vi "CryoCooler GUI.vi"(9 "Standalone":bool=TRUE, 10 "Init Data":variant, 11 "CryoCooler Name":string) -> ()   [LabVIEW 2024]
uses:
  typedefs/CC enum Operation Mode.ctl
  Cryo Cooler/CryoCoolerAVC/CryoCoolerAVC Command enum.ctl
  Subsystems/SS typedef cluster Instrument Command Queue Data.ctl
  Subsystems/SS cluster Data Queue type.ctl
  hk-channel-class/hk-channel-class/HK Item/HK Item.lvclass
  Cryo Cooler/Cryo Cooler.lvclass
  Cryo Cooler/CryoCoolerAVC/CryoCoolerAVC Command cluster.ctl
  typedefs/CC cluster Alarm Data.ctl
  CryoCooler cluster Alarm Settings.ctl
  Power Distribution/Power Distribution.lvclass
  typedefs/CC cluster Outlet Control.ctl
  typedefs/CC enum Status FG Action.ctl
  Cryo Cooler/CryoCoolerAVC/CryoCoolerAVC.lvclass
  typedefs/CC enum Subsystem Status.ctl
  hk-channel-class/hk-channel-class/HK Item/HK Item.lvclass/HK Item.ctl
  Power Distribution/Orion PDU/Orion PDU.lvclass
  hk-channel-class/hk-channel-class/HK Item/HK Channel cluster Telemetry Data.ctl
  hk-channel-class/hk-channel-class/HK Item/HK Channel enum Data Type.ctl
  <vilib>/Utility/error.llb/DialogType.ctl
  hk-channel-class/hk-channel-class/HK Item/Write Source.vi
  6db094d1-7fd6-4988-9962-decbce56bcaa.vi
  40afddd7-fa93-47ab-b467-3e4868690066.vi
panel:
  in  "Mode":T1
  in  "Tab Control":T2(tab)
  out "Alarm Message":string
  out "Cryo Connected":bool
  out "Alarm":bool
  in  "Status":i32[](listbox)
  out "XY Graph":T3(graph)
  out "Cryo 2":bool
  out "Cryo 1":bool
  in  "Configure Alarms":bool
  in  "Select Cryo Cooler":u16(ring) items=["Cooler1", "Cooler2", "Cooler3"]
  in  "Shutdown Temp":dbl caption="Reject Temp Shutdown Temp"
  in  "Init Message":string="Connecting to Hardware..."
  in  "Reinit":bool
  out "Response":string[](array[string])
  in  "Execute command":bool
  in  "Command Options":string="On"
  in  "Command":T4=1 items=["STATUS", "COOLER", "E", "ERROR", "KD", "KI", "KP", "LOGIN", "LOGOUT", "MODE", "P", "PWOUT", "SENSOR", "TC", "TEMP RJ", "TTARGET", "VERSION"]
  in  "Address":refnum<visa-resource-name>
  in  "CryoCooler Type":u16(ring) items=["Simulation", "RIMAS"]
  in  "Close":bool
  out "x-y":u32
  in  "Simulate":bool
  out "Current 2":dbl caption="Current" format="%_3g"
  out "Current":dbl format="%_3g"
  in  "Settings Button 2":bool
  in  "Refresh Button 2":bool
  in  "Names 2":string[](array[string])=["OutletA", "OutletB", "Lshore325", "Lshore218", "Lshore331", "PfeifferG", "Comms", "Motor"] caption="Names"
  in  "Relay Set 2":bool[](array[boolean]) caption="Set"
  out "Status 2":bool[](array[boolean]) caption="Status"
  in  "Settings Button":bool
  in  "Names":string[](array[string])=["MACIE", "Cryo1_3", "Cryo2", "Lesker", "Hg Argon", "Krypton", "Mercury", "Xenon"]
  in  "Relay Set":bool[](array[boolean]) caption="Set"
  out "Status":bool[](array[boolean])
  in  "Refresh Button":bool
  out "Log":string
  in  "Cryo 1 Pwr":bool
  in  "Cryo 2 Pwr":bool
  # "PDU 1"
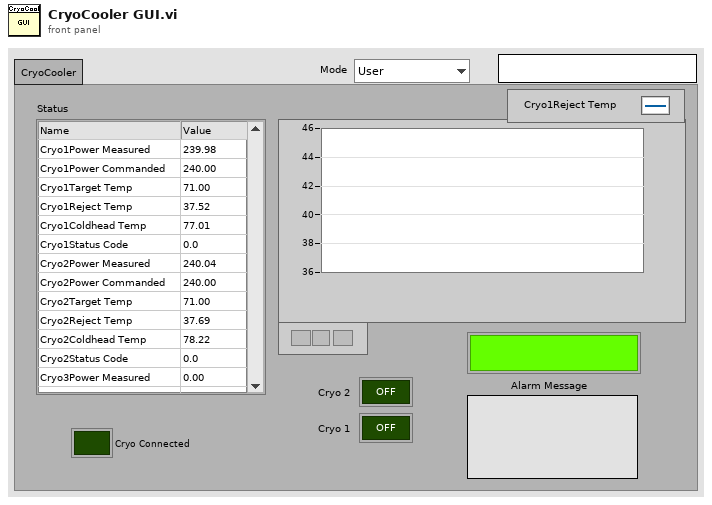
[diagram p1: front panel]
types:
  T1 = typedef "CC enum Operation Mode.ctl" = enum16{"User", "Engineering"}
  T2 = enum32{"CryoCooler", "Engineering", "Power", "Log"}
  T3 = cluster{cluster{"Time Stamp":timestamp, "Numeric":dbl}[]}[]
  T4 = typedef "CryoCoolerAVC.lvclass/CryoCoolerAVC Command enum.ctl" = u16
  T5 = typedef "SS typedef cluster Instrument Command Queue Data.ctl" = cluster{"Cmd":string, "Parameters":variant}
  T6 = typedef "CryoCoolerAVC.lvclass/CryoCoolerAVC Command cluster.ctl" = cluster{"Command":T4, "Options":string, "Cryo Idx":i32}
  T7 = typedef "CC cluster Alarm Data.ctl" = cluster{"Measured Value":dbl, "Alarm Low":dbl, "Alarm High":dbl, "Message":string, "Source":string}
  T8 = typedef "CryoCooler cluster Alarm Settings.ctl" = cluster{"Reject Shutdown Temp":dbl, "Reject Temp Warning":dbl, "Temperature Error Max":dbl, "Enabled":bool}
  T9 = typedef "CC cluster Outlet Control.ctl" = cluster{"Outlet Idx":i32, "State":bool}
  T10 = cluster{"state":refnum<user-event>, "cmd q":refnum<queue>, "Cmd":T5, "Data Q":refnum<queue>, "error":errorcluster, "next poll":timestamp, "Cryo Name":string, "poll":bool, "Channel List":refnum<class "HK Item.lvclass">[], "Focus Pos":dbl, "Cryo Cooler ref":refnum<class "Cryo Cooler.lvclass">, "Data":dbl[], "Cryo Cmd":T6, "Alarm":bool, "Alarms":T7[], "Source":string, "Cryo Alarms":T8, "Shutdown":bool, "Relays Enable":bool, "PDUs":refnum<class "Power Distribution.lvclass">[], "outlet":T9}
  T11 = typedef "CC enum Status FG Action.ctl" = enum16{"Read", "Write", "Init"}
  T12 = typedef "CC enum Subsystem Status.ctl" = enum16{"Unknown", "Ready", "Error"}
  T13 = typedef "SS cluster Data Queue type.ctl" = cluster{"Source":string, "Type":string, "Data":variant}
  T14 = typedef "HK Item.lvclass/HK Channel enum Data Type.ctl" = enum16{"Floating Point", "Integer", "Enum", "String", "Waveform", "File"}
  T15 = typedef "HK Item.lvclass/HK Channel cluster Telemetry Data.ctl" = cluster{"Ch Names":string[], "Ch Values":dbl[], "Timestamp":timestamp, "Data Type":T14}
  T16 = typedef "CC cluster Device Index.ctl" = cluster{"Device Type Name":string, "Curr Device Name":string, "All Instances":string[]}
  T17 = typedef "CryoCooler Default User Settings.ctl" = cluster{"Select Ch":i32[], "Default Device":string}
  T18 = typedef "CryoCoolerAVC.lvclass/CryoCoolerAVC Settings.ctl" = cluster{"Cryo Addr":refnum<visa-resource-name>[]}
  T19 = typedef "HK Item.lvclass/HK Channel Units and Setup.ctl" = cluster{"Unit Type":string, "Units":string, "Configuration":string, "Digits":i32, "Data Type":T14, "Exponential?":bool, "Source":string}
  T20 = cluster{"[0]":dbl, "[1]":dbl, "[2]":dbl, "[3]":dbl, "[4]":dbl, "[5]":dbl}[]
  T21 = cluster{cluster{"Time Stamp":timestamp, "Numeric":dbl}[]}
  T22 = typedef "DialogType.ctl" = u16
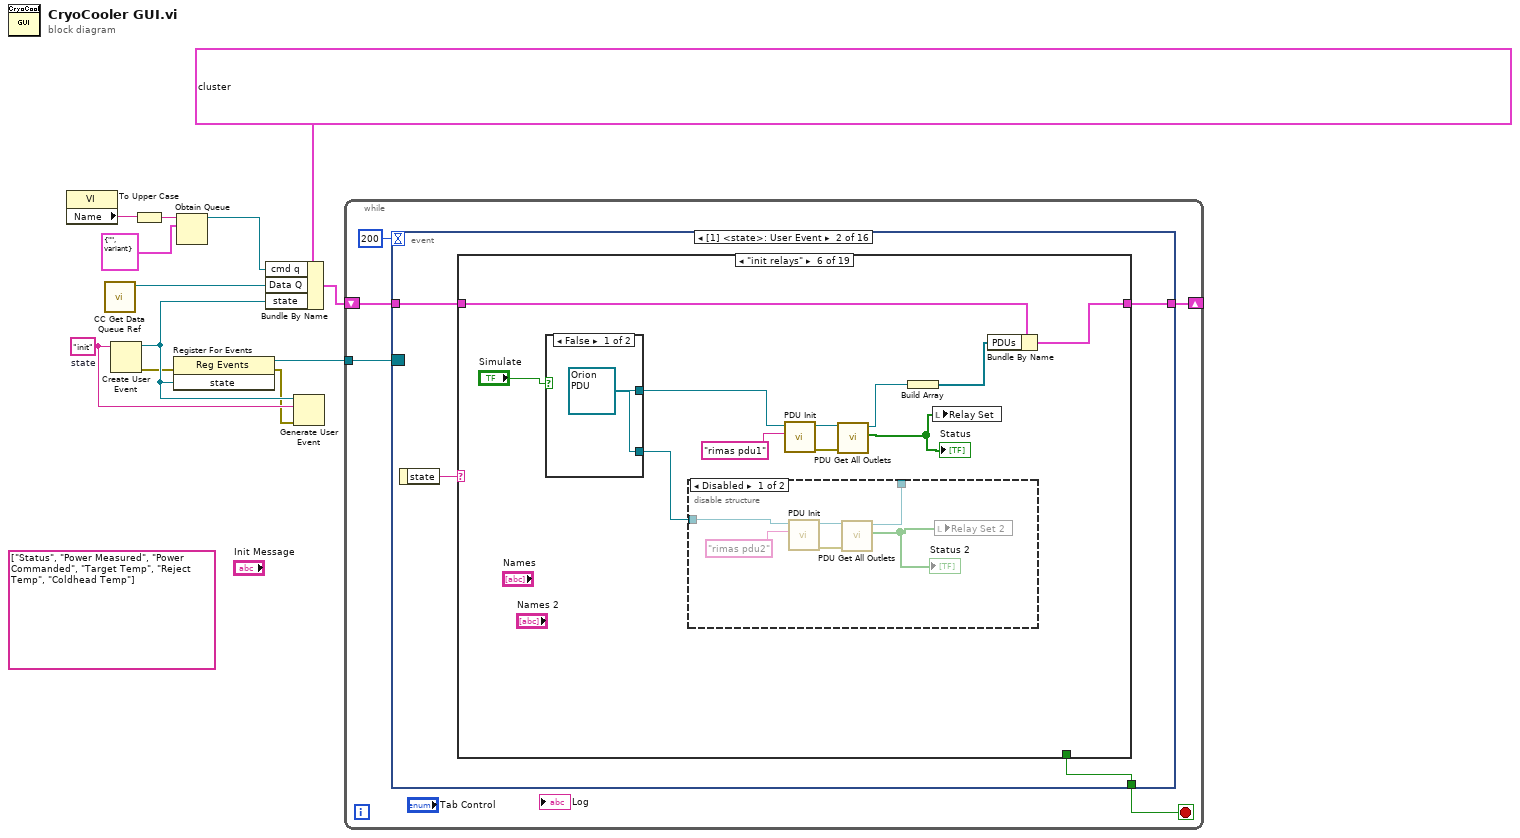
[diagram p0: block diagram]
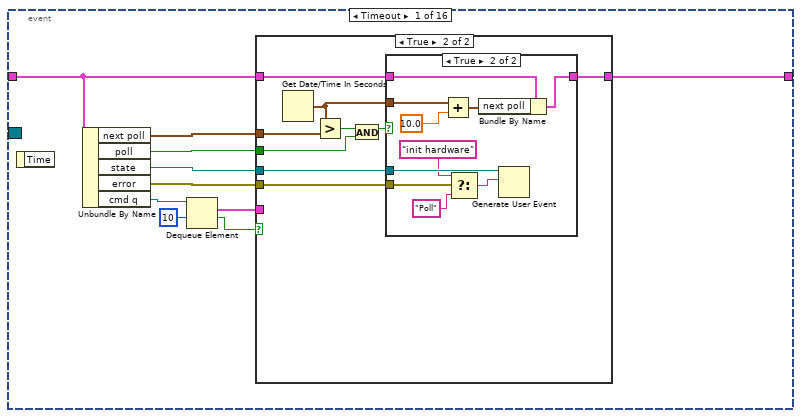
[diagram p2: hidden frame]
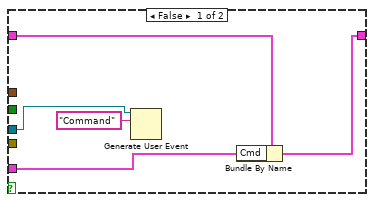
[diagram p3: hidden frame]
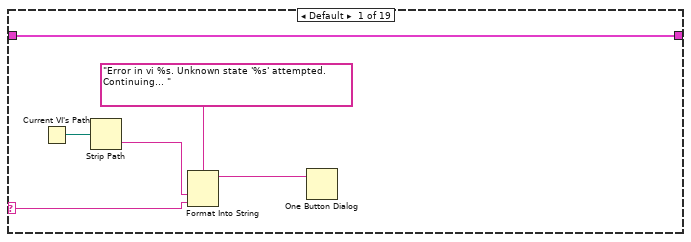
[diagram p5: hidden frame]
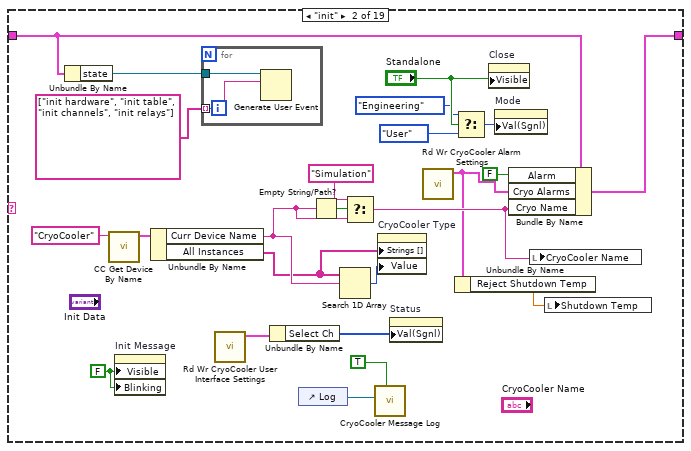
[diagram p6: hidden frame]
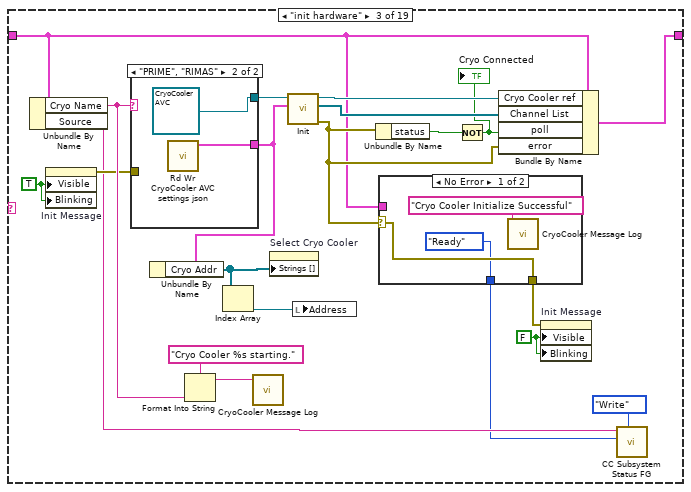
[diagram p7: hidden frame]
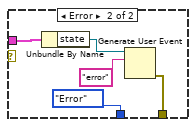
[diagram p8: hidden frame]
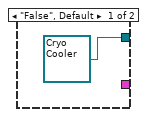
[diagram p9: hidden frame]
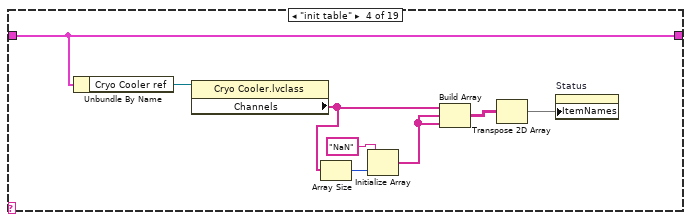
[diagram p10: hidden frame]
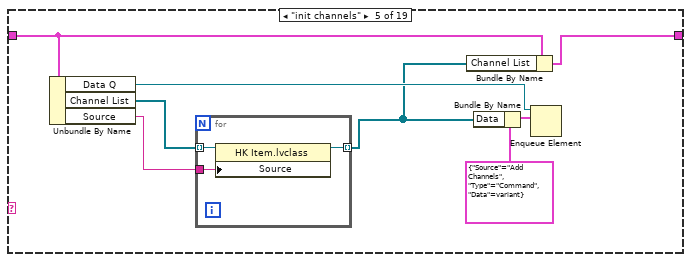
[diagram p11: hidden frame]
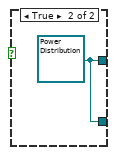
[diagram p13: hidden frame]
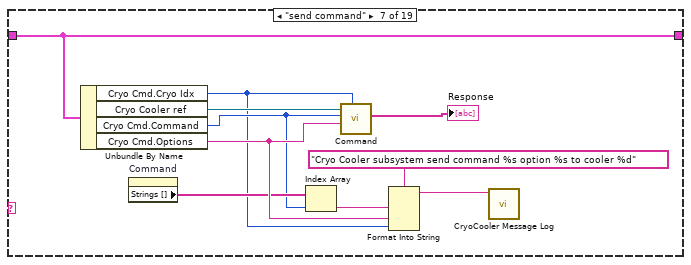
[diagram p14: hidden frame]
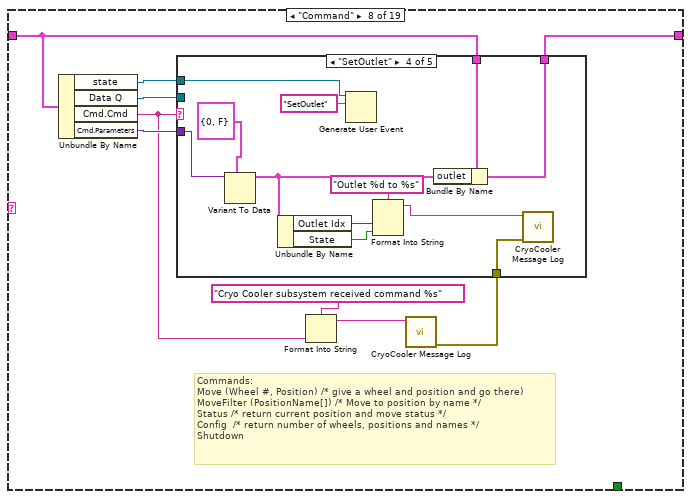
[diagram p15: hidden frame]
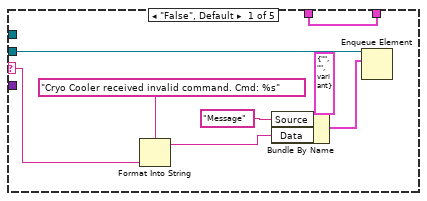
[diagram p16: hidden frame]
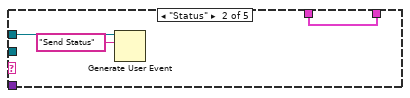
[diagram p17: hidden frame]
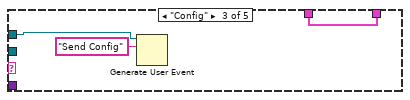
[diagram p18: hidden frame]
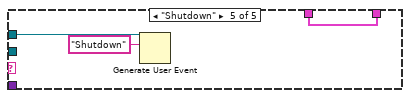
[diagram p19: hidden frame]
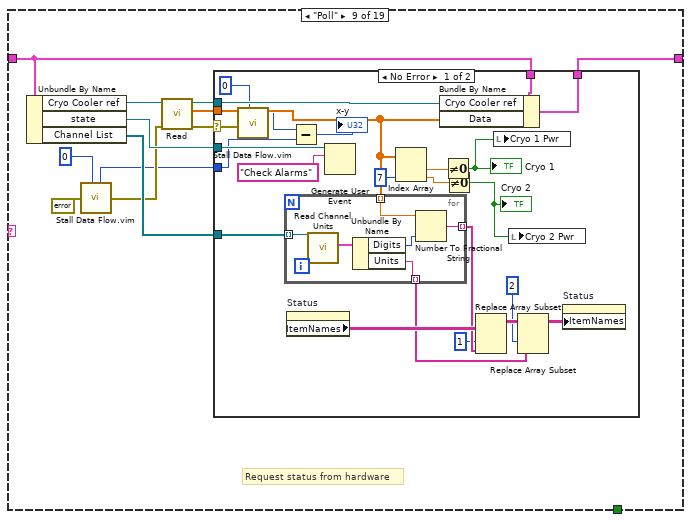
[diagram p20: hidden frame]
diagram:
  (unwired) string[] ["Status", "Power Measured", "Power Commanded", "Target Temp", "Reject Temp", "Coldhead Temp"]
  w8 = "init"  # state
  n1 = property class="VI"() -> ("Name"=w4:string)  [unwired: 2 in, 2 out]
  n2 = call "CC Get Data Queue Ref.vi"() -> ("Data Q"=w5:refnum<queue>)  [unwired: 10 in, 1 out]
  n3 = Create User Event(user event datatype=w8) -> (user event=w10:refnum<user-event>, error out=w6:errorcluster)  [unwired: 1 in]
  n4 = To Upper Case(1:w4) -> (0:w3:string)
  n5 = register-events(error in=w6, w10) -> (reference out=w9:refnum<event-registration>, error out=w7:errorcluster)  [unwired: 1 in]
  n6 = Obtain Queue(name (unnamed)=w3, element data type=T5 {"Cmd"="", "Parameters"=variant}) -> (queue out=w1:refnum<queue>)  [unwired: 3 in, 2 out]
  n7 = Bundle By Name(cluster=T10 {"state"=refnum, "cmd q"=refnum, "Cmd"={"Cmd"="", "Parameters"=variant}, "Data Q"=refnum, "error"={"status"=FALSE, "code"=0, "source"=""}, "next poll"=timestamp(0 s since 1904-01-01), "Cryo Name"="", "poll"=FALSE, "Channel List"=[], "Focus Pos"=0.0, "Cryo Cooler ref"=refnum, "Data"=[], "Cryo Cmd"={"Command"=0, "Options"="", "Cryo Idx"=0}, "Alarm"=FALSE, "Alarms"=[], "Source"="CryoCooler", "Cryo Alarms"={"Reject Shutdown Temp"=30.0, "Reject Temp Warning"=3.0, "Temperature Error Max"=60.0, "Enabled"=FALSE}, "Shutdown"=FALSE, "Relays Enable"=FALSE, "PDUs"=[], "outlet"={"Outlet Idx"=0, "State"=FALSE}}, "cmd q"=w1, "Data Q"=w5, "state"=w10) -> (w11:T10)
  n8 = Generate User Event(user event=w10, event data cluster=w8, error in=w7) -> ()  [unwired: 1 in, 2 out]
  n9 = while {
    tunnel: w9 -> [w17]
    shift-right: [w15] -> _
    shift-left: w11 -> [w16]
    stop <- w14 stop-if-true
    n10 = event shown="[1] <state>: User Event" {
      selector: w17 -> [_ _ _ _ _ _ _ _ _ _ _ _ _ _ _ _]
      dyn-events: _ -> [_ _ _ _ _ _ _ _ _ _ _ _ _ _ _ _]
      timeout: 200 -> [_ _ _ _ _ _ _ _ _ _ _ _ _ _ _ _]
      tunnel: w16 -> [w22 w55 w382 w397 w401 w409 w415 w425 w437 w451 w453 w459 w467 w473 w492 w499]
      tunnel: [w21 w54 w383 w398 w402 w407 w415 w425 w438 w451 w453 w460 w467 w474 w492 w499] -> w15
      tunnel: [_ w53 _ _ _ _ _ _ _ _ _ _ _ _ _ _] -> w14
      event Timeout {
        n11 = event-data() -> ()  [unwired: 1 in, 1 out]
        n12 = Unbundle By Name(w22) -> ("next poll"=w20:timestamp, "poll"=w19:bool, "state"=w23:refnum<user-event>, "error"=w18:errorcluster, "cmd q"=w27:refnum<queue>)
        n13 = Dequeue Element(queue=w27, timeout in ms (-1)=10) -> (element=w24:T5, timed out?=w25:bool)  [unwired: 1 in, 2 out]
        n14 = case shown="True" w25 {
          tunnel: w24 -> [w29 _]
          tunnel: w23 -> [w32 w38]
          tunnel: w22 -> [w30 w39]
          tunnel: [w28 w36] -> w21
          tunnel: w20 -> [_ w41]
          tunnel: w19 -> [_ w34]
          tunnel: w18 -> [_ w33]
          frame False {
            n15 = Generate User Event(user event=w32, event data cluster="Command" ("event data")) -> ()  [unwired: 2 in, 2 out]
            n16 = Bundle By Name(cluster=w30, "Cmd"=w29) -> (w28:T10)
          }
          frame True {
            n17 = Get Date/Time In Seconds() -> (seconds since 1Jan1904=w37:timestamp)
            n18 = Greater?(x=w37, y=w41) -> (0:w40:bool)
            n19 = And(x=w40, y=w34) -> (x .and. y?=w35:bool)
            n20 = case shown="True" w35 {
              tunnel: w39 -> [w42 w52]
              tunnel: w38 -> [_ w51]
              tunnel: w37 -> [_ w50]
              tunnel: [w42 w47] -> w36
              tunnel: w33 -> [_ w45]
              frame False {
              }
              frame True {
                n21 = Add(x=w50, y=10.0) -> (x+y=w48:timestamp)
                n22 = Select(t="init hardware", s=w45, f="Poll" ("event data")) -> (s? t:f=w43:string)
                n23 = Bundle By Name(cluster=w52, "next poll"=w48) -> (w47:T10)
                n24 = Generate User Event(user event=w51, event data cluster=w43) -> ()  [unwired: 2 in, 2 out]
              }
            }
          }
        }
      }
      event User Event {
        n25 = event-data() -> ("state"=w56:string)  [unwired: 1 in]
        n26 = case shown="\"init relays\"" w56 {
          selector: w56 -> [w61 _ _ _ _ _ _ _ _ _ _ _ _ _ _ _ _ _ _]
          tunnel: w55 -> [w57 w84 w100 w128 w130 w148 w167 w173 w217 w266 w280 w284 w297 w305 w317 w335 w339 w346 w371]
          tunnel: [w57 w85 w109 w128 w131 w150 w167 w174 w218 w267 w280 w285 w297 w305 w317 w335 w340 w347 w371] -> w54
          tunnel: [_ _ _ _ _ _ _ _ _ _ _ _ _ _ _ _ _ _ TRUE] -> w53
          frame Default {
            n27 = Current VI's Path() -> (path=w60:path)
            n28 = Strip Path(path=w60) -> (name=w59:string)  [unwired: 1 out]
            n29 = Format Into String(format string="Error in vi %s. Unknown state '%s' attempted. Continuing... ", w59, w61) -> (resulting string=w58:string)  [unwired: 2 in, 1 out]
            n30 = One Button Dialog(message=w58) -> ()  [unwired: 1 in, 1 out]
          }
          frame "init" {
            w66 = FALSE ("Visible")
            n31 = Unbundle By Name(w84) -> ("state"=w83:refnum<user-event>)
            n32 = call "CC Get Device By Name.vi"("Device Type"="CryoCooler") -> ("Device"=w78:T16)  [unwired: 8 in, 2 out]
            n33 = property on="Init Message" class="Str"("Visible"=w66, "Blinking"=w66) -> ()  [unwired: 2 in, 2 out]
            n34 = Unbundle By Name(w78) -> ("Curr Device Name"=w77:string, "All Instances"=w76:string[])
            n35 = for {
              tunnel: w83 -> [w88]
              tunnel: string[] ["init hardware", "init table", "init channels", "init relays"] -> [w87] mode=indexing
              n36 = Generate User Event(user event=w88, event data cluster=w87) -> ()  [unwired: 2 in, 2 out]
            }
            n37 = call "Rd Wr CryoCooler User Interface Settings.vi"() -> ("Settings"=w71:T17)  [unwired: 10 in, 1 out]
            n38 = Unbundle By Name(w71) -> ("Select Ch"=w70:i32[])
            n39 = control-ref of="Log"() -> (w69:refnum<vi>)
            n40 = Empty String/Path?(string/path=w77) -> (empty?=w86:bool)
            n41 = Search 1D Array(1D array=w76, element=w77) -> (index of element=w81:i32)  [unwired: 1 in]
            n42 = Select(t="Simulation", s=w86, f=w77) -> (s? t:f=w67:string)
            n43 = call "CryoCooler Message Log.vi"("init?"=TRUE, "Log Ref"=w69) -> ()  [unwired: 8 in, 2 out]
            n44 = property on="CryoCooler Type" class="Ring (strict)"("Strings []"=w76, "Value"=w81) -> ()  [unwired: 2 in, 2 out]
            n45 = property on="Status" class="MCListbox (strict)"("Val(Sgnl)"=w70) -> ()  [unwired: 2 in, 2 out]
            n46 = call "Rd Wr CryoCooler Alarm Settings.vi"() -> ("Cryo Alarms out"=w65:T8)  [unwired: 10 in, 1 out]
            n47 = Unbundle By Name(w65) -> ("Reject Shutdown Temp"=w64:dbl)
            n48 = Select(t=CC_enum_Operation_Mode."Engineering" ("Mode"), s="Standalone", f=CC_enum_Operation_Mode."User" ("Mode")) -> (s? t:f=w72:T1)
            n49 = property on="Close" class="Bool"("Visible"="Standalone") -> ()  [unwired: 2 in, 2 out]
            n50 = property on="Mode" class="Enum (strict)"("Val(Sgnl)"=w72) -> ()  [unwired: 2 in, 2 out]
            n51 = Bundle By Name(cluster=w84, "Alarm"=FALSE, "Cryo Alarms"=w65, "Cryo Name"=w67) -> (w85:T10)
            n52 = local write "CryoCooler Name"(w67) -> ()
            n53 = local write "Shutdown Temp"(w64) -> ()
          }
          frame "init hardware" {
            w95 = FALSE ("Visible")
            w97 = TRUE ("Visible")
            n54 = Unbundle By Name(w100) -> ("Cryo Name"=w104:string, "Source"=w92:string)
            n55 = property on="Init Message" class="Str"("Visible"=w97, "Blinking"=w97) -> (error out=w96:errorcluster)  [unwired: 2 in, 1 out]
            n56 = case shown="\"PRIME\", \"RIMAS\"" w104 {
              tunnel: [refnum<class "Cryo Cooler.lvclass"> refnum ("Cryo Cooler.lvclass") refnum<class "CryoCoolerAVC.lvclass"> refnum ("CryoCoolerAVC.lvclass")] -> w106
              tunnel: [_ w119] -> w103
              tunnel: w96 -> [_ _]
              frame "False", Default {
              }
              frame "PRIME", "RIMAS" {
                n57 = call "Rd Wr CryoCooler AVC settings json.vi"() -> ("CryoCooler Settings"=w119:T18)  [unwired: 10 in, 1 out]
              }
            }
            n58 = Unbundle By Name(w103) -> ("Cryo Addr"=w90:refnum<visa-resource-name>[])
            n59 = Format Into String(format string="Cryo Cooler %s starting.", w104) -> (resulting string=w98:string)  [unwired: 2 in, 1 out]
            n60 = Index Array(array=w90) -> (element=w89:refnum<visa-resource-name>)  [unwired: 1 in]
            n61 = call "CryoCooler Message Log.vi"("String in"=w98) -> ()  [unwired: 9 in, 2 out]
            n62 = property on="Select Cryo Cooler" class="Ring (strict)"("Strings []"=w90) -> ()  [unwired: 2 in, 2 out]
            n63 = call-dynamic "Init.vi"("Init Data"=w103, "Cryo Cooler in"=w106) -> ("error out"=w101:errorcluster, "Channel List"=w105:refnum<class "HK Item.lvclass">[], "Cryo Cooler out"=w107:refnum<class "Cryo Cooler.lvclass">)  [unwired: 7 in]
            n64 = local write "Address"(w89) -> ()
            n65 = Unbundle By Name(w101) -> ("status"=w108:bool)
            n66 = case shown="No Error" w101 {
              selector: w101 -> [w111 _]
              tunnel: w100 -> [_ w117]
              tunnel: [w111 w114] -> w94
              tunnel: [CC_enum_Subsystem_Status."Ready" ("Status") CC_enum_Subsystem_Status."Error" ("Status")] -> w91
              frame No Error {
                n67 = call "CryoCooler Message Log.vi"("String in"="Cryo Cooler Initialize Successful") -> ()  [unwired: 9 in, 2 out]
              }
              frame Error {
                n68 = Unbundle By Name(w117) -> ("state"=w116:refnum<user-event>)
                n69 = Generate User Event(user event=w116, event data cluster="error" ("event data")) -> (error out=w114:errorcluster)  [unwired: 2 in, 1 out]
              }
            }
            n70 = Not(x=w108) -> (.not. x?=w99:bool)
            "Cryo Connected" <- w99
            n71 = Bundle By Name(cluster=w100, "Cryo Cooler ref"=w107, "Channel List"=w105, "poll"=w99, "error"=w101) -> (w109:T10)
            n72 = property on="Init Message" class="Str"(error in=w94, "Visible"=w95, "Blinking"=w95) -> ()  [unwired: 1 in, 2 out]
            n73 = call "CC Subsystem Status FG.vi"("Action"=CC_enum_Status_FG_Action."Write", "Status"=w91, "Subsystem Name"=w92) -> ()  [unwired: 7 in, 2 out]
          }
          frame "init table" {
            n74 = Unbundle By Name(w128) -> ("Cryo Cooler ref"=w127:refnum<class "Cryo Cooler.lvclass">)
            n75 = property class="Cryo Cooler.lvclass"(reference=w127) -> ("Channels"=w125:string[])  [unwired: 1 in, 2 out]
            n76 = Array Size(array=w125) -> (size(s)=w126:i32)
            n77 = Initialize Array("NaN", w126) -> (w121:string[])
            n78 = Build Array(w125, w121, w121) -> (w123:string[][])
            n79 = Transpose 2D Array(2D array=w123) -> (transposed array=w122:string[][])
            n80 = property on="Status" class="MCListbox (strict)"("ItemNames"=w122) -> ()  [unwired: 2 in, 2 out]
          }
          frame "init channels" {
            n81 = Unbundle By Name(w130) -> ("Data Q"=w134:refnum<queue>, "Channel List"=w133:refnum<class "HK Item.lvclass">[], "Source"=w129:string)
            n82 = for {
              tunnel: w133 -> [w139] mode=indexing
              tunnel: [w138] -> w132 mode=indexing
              tunnel: w129 -> [w137]
              n83 = property class="HK Item.lvclass"(reference=w139, "Source"=w137) -> (reference out=w138:refnum<class "HK Item.lvclass">)  [unwired: 1 in, 1 out]
            }
            n84 = Bundle By Name(cluster=w130, "Channel List"=w132) -> (w131:T10)
            n85 = Bundle By Name(cluster=T13 {"Source"="Add Channels", "Type"="Command", "Data"=variant} ("element"), "Data"=w132) -> (w136:T13)
            n86 = Enqueue Element(queue=w134, element=w136) -> ()  [unwired: 2 in, 3 out]
          }
          frame "init relays" {
            n87 = case shown="False" "Simulate" {
              tunnel: [w157 w158] -> w145
              tunnel: [w157 w158] -> w141
              frame False {
                w157 = refnum<class "Orion PDU.lvclass"> refnum ("Orion PDU.lvclass")
              }
              frame True {
                w158 = refnum<class "Power Distribution.lvclass"> refnum ("PDU")
              }
            }
            n88 = disable-structure shown="Disabled" {
              disable-tunnel: [w153 _] -> _
              disable-tunnel: w141 -> [w151 _]
              frame Disabled {
                n89 = call-dynamic "PDU Init.vi"("Name"="rimas pdu2", "Power Distribution in"=w151) -> ("error out"=w155:errorcluster, "Power Distribution out"=w154:refnum<class "Power Distribution.lvclass">)  [unwired: 8 in]
                n90 = call-dynamic "PDU Get All Outlets.vi"("error in (no error)"=w155, "Power Distribution in"=w154) -> ("States"=w152:bool[], "Power Distribution out"=w153:refnum<class "Power Distribution.lvclass">)  [unwired: 6 in, 2 out]
                "Status 2" <- w152
                n91 = local write "Relay Set 2"(w152) -> ()
              }
              frame Enabled {
              }
            }
            n92 = call-dynamic "PDU Init.vi"("Name"="rimas pdu1", "Power Distribution in"=w145) -> ("error out"=w146:errorcluster, "Power Distribution out"=w149:refnum<class "Power Distribution.lvclass">)  [unwired: 8 in]
            n93 = call-dynamic "PDU Get All Outlets.vi"("error in (no error)"=w146, "Power Distribution in"=w149) -> ("States"=w147:bool[], "Power Distribution out"=w143:refnum<class "Power Distribution.lvclass">)  [unwired: 6 in, 2 out]
            "Status" <- w147
            n94 = Build Array(w143) -> (w142:refnum<class "Power Distribution.lvclass">[])
            n95 = local write "Relay Set"(w147) -> ()
            n96 = Bundle By Name(cluster=w148, "PDUs"=w142) -> (w150:T10)
          }
          frame "send command" {
            n97 = Unbundle By Name(w167) -> ("Cryo Cmd.Cryo Idx"=w159:i32, "Cryo Cooler ref"=w168:refnum<class "Cryo Cooler.lvclass">, "Cryo Cmd.Command"=w161:T4, "Cryo Cmd.Options"=w163:string)
            n98 = property on="Command" class="Ring (strict)"() -> ("Strings []"=w162:string[])  [unwired: 2 in, 2 out]
            n99 = Index Array(array=w162, index=w161) -> (element=w160:string)
            n100 = call-dynamic "Command.vi"("Cryo Idx"=w159, "Options"=w163, "Command"=w161, "Cryo Cooler in"=w168) -> ("Response"=→"Response":string[])  [unwired: 5 in, 2 out]
            n101 = Format Into String(format string="Cryo Cooler subsystem send command %s option %s to cooler %d", w160, w163, w159) -> (resulting string=w164:string)  [unwired: 2 in, 1 out]
            n102 = call "CryoCooler Message Log.vi"("String in"=w164) -> ()  [unwired: 9 in, 2 out]
          }
          frame "Command" {
            # "Commands:\nMove (Wheel #, Position) /* give a wheel and position and go there)\nMoveFilter (PositionName[]) /* Move to position by name */\nStatus /* return current position and move status */\nConfig  /* return number of wheels, positions and names */\nShutdown"
            n103 = Unbundle By Name(w173) -> ("state"=w175:refnum<user-event>, "Data Q"=w177:refnum<queue>, "Cmd.Cmd"=w171:string, "Cmd.Parameters"=w176:variant)
            n104 = Format Into String(format string="Cryo Cooler subsystem received command %s", w171) -> (resulting string=w170:string)  [unwired: 2 in, 1 out]
            n105 = call "CryoCooler Message Log.vi"("String in"=w170) -> ("error out"=w169:errorcluster)  [unwired: 9 in, 1 out]
            n106 = case shown="\"SetOutlet\"" w171 {
              selector: w171 -> [w179 _ _ _ _]
              tunnel: w177 -> [w185 _ _ _ _]
              tunnel: w176 -> [_ _ _ w201 _]
              tunnel: w175 -> [_ w188 w190 w202 w206]
              tunnel: w173 -> [w178 w186 w189 w200 w204]
              tunnel: [w178 w186 w189 w199 w204] -> w174
              tunnel: w169 -> [_ _ _ w197 _]
              frame "False", Default {
                n107 = Format Into String(format string="Cryo Cooler received invalid command. Cmd: %s", w179) -> (resulting string=w181:string)  [unwired: 2 in, 1 out]
                n108 = Bundle By Name(cluster=T13 {"Source"="", "Type"="", "Data"=variant} ("element"), "Source"="Message" ("Data Type"), "Data"=w181) -> (w180:T13)
                n109 = Enqueue Element(queue=w185, element=w180) -> ()  [unwired: 2 in, 3 out]
              }
              frame "Status" {
                n110 = Generate User Event(user event=w188, event data cluster="Send Status" ("event data")) -> ()  [unwired: 2 in, 2 out]
              }
              frame "Config" {
                n111 = Generate User Event(user event=w190, event data cluster="Send Config" ("event data")) -> ()  [unwired: 2 in, 2 out]
              }
              frame "SetOutlet" {
                n112 = Variant To Data(type=T9 {"Outlet Idx"=0, "State"=FALSE} ("outlet parm in"), Variant=w201) -> (data=w195:T9)  [unwired: 1 in, 1 out]
                n113 = Unbundle By Name(w195) -> ("Outlet Idx"=w194:i32, "State"=w193:bool)
                n114 = Generate User Event(user event=w202, event data cluster="SetOutlet" ("event data")) -> ()  [unwired: 2 in, 2 out]
                n115 = Format Into String(format string="Outlet %d to %s", w194, w193) -> (resulting string=w192:string)  [unwired: 2 in, 1 out]
                n116 = Bundle By Name(cluster=w200, "outlet"=w195) -> (w199:T10)
                n117 = call "CryoCooler Message Log.vi"("error in (no error)"=w197, "String in"=w192) -> ()  [unwired: 8 in, 2 out]
              }
              frame "Shutdown" {
                n118 = Generate User Event(user event=w206, event data cluster="Shutdown" ("event data")) -> ()  [unwired: 2 in, 2 out]
              }
            }
          }
          frame "Poll" {
            # "Request status from hardware"
            n119 = Unbundle By Name(w217) -> ("Cryo Cooler ref"=w215:refnum<class "Cryo Cooler.lvclass">, "state"=w216:refnum<user-event>, "Channel List"=w213:refnum<class "HK Item.lvclass">[])
            n120 = call "Stall Data Flow.vim"("value in"=errorcluster {"status"=FALSE, "code"=0, "source"=""} ("error in (no error)"), "milliseconds to wait"=u32 0) -> ("millisecond timer value"=w207:u32, "value out"=w209:errorcluster)
            n121 = call-dynamic "Read.vi"("error in (no error)"=w209, "Cryo Cooler in"=w215) -> ("error out"=w211:errorcluster, "Data"=w212:dbl[], "Cryo Cooler out"=w214:refnum<class "Cryo Cooler.lvclass">)  [unwired: 7 in]
            n122 = case shown="No Error" w211 {
              selector: w211 -> [w229 w250]
              tunnel: [w242 w249] -> w218
              tunnel: w217 -> [w241 w251]
              tunnel: w216 -> [w240 w253]
              tunnel: w214 -> [w238 _]
              tunnel: w213 -> [w237 _]
              tunnel: w212 -> [w236 _]
              tunnel: w207 -> [w226 _]
              frame No Error {
                n123 = call "Stall Data Flow.vim"("value in"=w229, "milliseconds to wait"=u32 0) -> ("millisecond timer value"=w227:u32)  [unwired: 1 out]
                n124 = for {
                  tunnel: w237 -> [w248] mode=indexing
                  tunnel: w236 -> [w245] mode=indexing
                  tunnel: [w244] -> w233 mode=indexing
                  tunnel: [w243] -> w220 mode=indexing
                  n125 = call "Read Channel Units.vi"("HK Item in"=w248) -> ("Channel Setup"=w247:T19)  [unwired: 8 in, 2 out]
                  n126 = Unbundle By Name(w247) -> ("Digits"=w246:i32, "Units"=w243:string)
                  n127 = Number To Fractional String(number=w245, precision (6)=w246) -> (F-format string=w244:string)  [unwired: 2 in]
                }
                n128 = property on="Status" class="MCListbox (strict)"() -> ("ItemNames"=w234:string[][])  [unwired: 2 in, 2 out]
                n129 = Subtract(x=w227, y=w226) -> (x-y=→"x-y":u32)
                n130 = Generate User Event(user event=w240, event data cluster="Check Alarms" ("event data")) -> ()  [unwired: 2 in, 2 out]
                n131 = Index Array(array=w236, index #2=7 ("index")) -> (element #1=w235:dbl, element #2=w230:dbl)  [unwired: 1 in]
                n132 = Bundle By Name(cluster=w241, "Cryo Cooler ref"=w238, "Data"=w236) -> (w242:T10)
                n133 = Not Equal To 0?(x=w235) -> (x != 0?=w224:bool)
                "Cryo 1" <- w224
                n134 = Not Equal To 0?(x=w230) -> (x != 0?=w223:bool)
                "Cryo 2" <- w223
                n135 = Replace Array Subset(array=w234, new element=w233, index (col)=1 ("disabled index (col)")) -> (w222:string[][])  [unwired: 1 in]
                n136 = local write "Cryo 1 Pwr"(w224) -> ()
                n137 = local write "Cryo 2 Pwr"(w223) -> ()
                n138 = Replace Array Subset(array=w222, new element=w220, index (col)=2 ("disabled index (col)")) -> (w219:string[][])  [unwired: 1 in]
                n139 = property on="Status" class="MCListbox (strict)"("ItemNames"=w219) -> ()  [unwired: 2 in, 2 out]
              }
              frame Error {
                n140 = Generate User Event(user event=w253, event data cluster="error" ("event data")) -> ()  [unwired: 2 in, 2 out]
                n141 = Bundle By Name(cluster=w251, "error"=w250) -> (w249:T10)
              }
            }
          }
          frame "Check Alarms" {
            n142 = Unbundle By Name(w266) -> ("state"=w257:refnum<user-event>, "Data"=w255:dbl[], "Alarm"=w261:bool, "Cryo Alarms"=w260:T8, "Shutdown"=w259:bool)
            n143 = call "Data Array to Cluster.vi"("Data"=w255) -> ("Data out"=w254:T20)  [unwired: 10 in]
            n144 = Generate User Event(user event=w257, event data cluster="Read PDU" ("event data")) -> ()  [unwired: 2 in, 2 out]
            n145 = call "CryoCooler Alarm Check.vi"("Cryo Alarms"=w260, "Array"=w254) -> ("shutdown?"=w256:bool, "Alarms"=w264:T7[], "Alarm"=w262:bool)  [unwired: 6 in, 1 out]
            "Alarm" <- w262
            n146 = Compound Arithmetic op=AND(w262, invert w261) -> (w265:bool)
            n147 = Compound Arithmetic op=AND(w261, invert w262) -> (w263:bool)
            n148 = Compound Arithmetic op=AND(w256, invert w259) -> (w258:bool)
            n149 = case shown="True" w265 {
              tunnel: w257 -> [_ w274]
              frame False {
              }
              frame True {
                n150 = Generate User Event(user event=w274, event data cluster="Alarm Set" ("event data")) -> ()  [unwired: 2 in, 2 out]
              }
            }
            n151 = case shown="True" w263 {
              tunnel: w257 -> [_ w272]
              frame False {
              }
              frame True {
                n152 = Generate User Event(user event=w272, event data cluster="Alarm Clear" ("event data")) -> ()  [unwired: 2 in, 2 out]
              }
            }
            n153 = case shown="True" w258 {
              tunnel: w257 -> [_ w270]
              frame False {
              }
              frame True {
                n154 = Generate User Event(user event=w270, event data cluster="Alarm Shutdown" ("event data")) -> ()  [unwired: 2 in, 2 out]
              }
            }
            n155 = Bundle By Name(cluster=w266, "Shutdown"=w256, "Alarm"=w262, "Alarms"=w264) -> (w267:T10)
          }
          frame "Read PDU" {
            n156 = Unbundle By Name(w280) -> ("state"=w279:refnum<user-event>, "PDUs"=w278:refnum<class "Power Distribution.lvclass">[])
            n157 = for {
              tunnel: w278 -> [w283] mode=indexing
              tunnel: [w282] -> w277 mode=indexing
              n158 = call-dynamic "PDU Get All Outlets.vi"("Power Distribution in"=w283) -> ("current"=w282:dbl)  [unwired: 7 in, 3 out]
            }
            n159 = Generate User Event(user event=w279, event data cluster="Send Status" ("event data")) -> ()  [unwired: 2 in, 2 out]
            n160 = Index Array(array=w277) -> (element #1=→"Current":dbl, element #2=→"Current 2":dbl)  [unwired: 2 in]
          }
          frame "SetOutlet" {
            n161 = Unbundle By Name(w284) -> ("PDUs"=w289:refnum<class "Power Distribution.lvclass">[], "outlet.Outlet Idx"=w291:i32, "outlet.State"=w290:bool)
            n162 = Index Array(array=w289) -> (element=w292:refnum<class "Power Distribution.lvclass">)  [unwired: 1 in]
            n163 = call-dynamic "PDU Set By Index.vi"("state"=w290, "Index"=w291, "Power Distribution in"=w292) -> ("Power Distribution out"=w288:refnum<class "Power Distribution.lvclass">)  [unwired: 7 in, 1 out]
            n164 = Replace Array Subset(array=w289, new element=w288, index=0) -> (w286:refnum<class "Power Distribution.lvclass">[])
            n165 = Bundle By Name(cluster=w284, "PDUs"=w286) -> (w285:T10)
          }
          frame "Alarm Set" {
            n166 = Unbundle By Name(w297) -> ("Data Q"=w302:refnum<queue>, "Source"=w294:string, "Alarms"=w299:T7[])
            n167 = Index Array(array=w299) -> (element=w298:T7)  [unwired: 1 in]
            n168 = Bundle By Name(cluster=w298, "Source"=w294) -> (w295:T7)
            n169 = Unbundle By Name(w295) -> ("Message"=w296:string)
            "Alarm Message" <- w296
            n170 = Bundle By Name(cluster=T13 {"Source"="", "Type"="", "Data"=variant} ("element"), "Source"=w294, "Type"="Alarm Set", "Data"=w295) -> (w293:T13)
            n171 = Enqueue Element(queue=w302, element=w293) -> ()  [unwired: 2 in, 3 out]
            n172 = call "CryoCooler Message Log.vi"("String in"=w296) -> ()  [unwired: 9 in, 2 out]
          }
          frame "Alarm Clear" {
            n173 = Unbundle By Name(w305) -> ("Data Q"=w309:refnum<queue>, "Source"=w306:string)
            n174 = Bundle By Name(cluster=T13 {"Source"="", "Type"="", "Data"=variant} ("element"), "Source"=w306, "Type"="Alarm Clear") -> (w303:T13)
            n175 = call "CryoCooler Message Log.vi"("String in"="Alarm condition cleared.") -> ()  [unwired: 9 in, 2 out]
            n176 = Enqueue Element(queue=w309, element=w303) -> ()  [unwired: 2 in, 3 out]
          }
          frame "Alarm Shutdown" {
            w312 = "Off"
            w311 = T4 1 items=["STATUS", "COOLER", "E", "ERROR", "KD", "KI", "KP", "LOGIN", "LOGOUT", "MODE", "P", "PWOUT", "SENSOR", "TC", "TEMP RJ", "TTARGET", "VERSION"] ("Cryo Cmd.Command")
            n177 = Unbundle By Name(w317) -> ("Cryo Cooler ref"=w318:refnum<class "Cryo Cooler.lvclass">)
            n178 = call-dynamic "Command.vi"("Cryo Idx"=0, "Options"=w312, "Command"=w311, "Cryo Cooler in"=w318) -> ("error out"=w310:errorcluster, "Cryo Cooler out"=w315:refnum<class "Cryo Cooler.lvclass">)  [unwired: 5 in, 1 out]
            n179 = call-dynamic "Command.vi"("Cryo Idx"=1, "error in (no error)"=w310, "Options"=w312, "Command"=w311, "Cryo Cooler in"=w315) -> ()  [unwired: 4 in, 3 out]
            n180 = call "CryoCooler Message Log.vi"("String in"="Cryo Cooler reject temperature too high. Turning off Cryo Coolers.") -> ()  [unwired: 9 in, 2 out]
          }
          frame "Send Status" {
            n181 = Unbundle By Name(w335) -> ("Data Q"=w334:refnum<queue>, "Source"=w319:string, "Cryo Cooler ref"=w327:refnum<class "Cryo Cooler.lvclass">, "Data"=w324:dbl[])
            n182 = Get Date/Time In Seconds() -> (seconds since 1Jan1904=w325:timestamp)
            n183 = call-dynamic "Read Channels.vi"("Cryo Cooler in"=w327) -> ("Channels"=w326:string[])  [unwired: 8 in, 2 out]
            n184 = Bundle(cluster=T15 {"Ch Names"=[], "Ch Values"=[], "Timestamp"=timestamp(0 s since 1904-01-01), "Data Type"=enum."Floating Point"}, "Ch Names"=w326, "Ch Values"=w324, "Timestamp"=w325, "Data Type"=HK_Channel_enum_Data_Type."Floating Point") -> (w329:T15)
            n185 = call "CC CryoCooler Data buffer.vi"("Write?"=TRUE, "Data"=w324, "Time Stamp"=w325) -> ("XY Graph"=w321:T3)  [unwired: 7 in, 1 out]
            n186 = for {
              tunnel: "Status" -> [w337] mode=indexing
              tunnel: w321 -> [w338]
              tunnel: [w336] -> w320 mode=indexing
              n187 = Index Array(array=w338, index=w337) -> (element=w336:T21)
            }
            "XY Graph" <- w320
            n188 = Bundle By Name(cluster=T13 {"Source"="", "Type"="", "Data"=variant} ("element"), "Source"=w319, "Type"="Floating Point" ("Data Type"), "Data"=w329) -> (w331:T13)
            n189 = Enqueue Element(queue=w334, element=w331) -> ()  [unwired: 2 in, 3 out]
          }
          frame "Reinit" {
            n190 = Unbundle By Name(w339) -> ("Cryo Cooler ref"=w343:refnum<class "Cryo Cooler.lvclass">, "state"=w345:refnum<user-event>)
            n191 = call-dynamic "Close.vi"("Cryo Cooler in"=w343) -> ("error out"=w342:errorcluster, "Cryo Cooler out"=w341:refnum<class "Cryo Cooler.lvclass">)  [unwired: 9 in]
            n192 = Generate User Event(user event=w345, event data cluster="init hardware" ("event data")) -> ()  [unwired: 2 in, 2 out]
            n193 = call <vilib>:"Clear Errors.vi"("error in (no error)"=w342) -> ()  [unwired: 5 in, 2 out]
            n194 = Bundle By Name(cluster=w339, "Cryo Cooler ref"=w341) -> (w340:T10)
          }
          frame "error" {
            w359 = T22 0 items=["no dialog", "OK message", "continue or stop message", "OK message + warnings", "continue/stop + warnings"] ("type of dialog (OK msg:1)")
            n195 = Unbundle By Name(w346) -> ("Cryo Name"=w351:string, "error"=w362:errorcluster, "error.code"=w365:i32, "error.source"=w363:string, "Data Q"=w353:refnum<queue>)
            n196 = call <vilib>:"Simple Error Handler.vi"("type of dialog (OK msg:1)"=w359, "error in (no error)"=w362) -> ("message"=w361:string)  [unwired: 3 in, 4 out]
            n197 = Bundle By Name(cluster=T7 {"Measured Value"=0.0, "Alarm Low"=0.0, "Alarm High"=0.0, "Message"="", "Source"=""} ("element"), "Source"=w351, "Message"="CryoCooler Initialization Error. Check Communications port.") -> (w355:T7)
            n198 = Format Into String(format string="Error from Cryo Cooler \"%s\". Error # %d, Error Source: %s, Error message \"%s\"", w351, w365, w363, w361) -> (resulting string=w360:string)  [unwired: 2 in, 1 out]
            n199 = Bundle By Name(cluster=T13 {"Source"="", "Type"="", "Data"=variant} ("element"), "Source"=w351, "Type"="Alarm Set", "Data"=w355) -> (w352:T13)
            n200 = call "CryoCooler Message Log.vi"("String in"=w360) -> ()  [unwired: 9 in, 2 out]
            n201 = Get Date/Time In Seconds() -> (seconds since 1Jan1904=w350:timestamp)
            n202 = Add(x=w350, y=120.0) -> (x+y=w348:timestamp)
            n203 = Enqueue Element(queue=w353, element=w352) -> ()  [unwired: 2 in, 3 out]
            n204 = Bundle By Name(cluster=w346, "next poll"=w348) -> (w347:T10)
          }
          frame "Shutdown" {
            n205 = Unbundle By Name(w371) -> ("Data Q"=w370:refnum<queue>, "Cryo Cooler ref"=w369:refnum<class "Cryo Cooler.lvclass">, "PDUs"=w366:refnum<class "Power Distribution.lvclass">[])
            n206 = for {
              tunnel: w366 -> [w373] mode=indexing
              n207 = call-dynamic "PDU Close.vi"("Power Distribution in"=w373) -> ()  [unwired: 9 in, 2 out]
            }
            n208 = call-dynamic "Close.vi"("Cryo Cooler in"=w369) -> ("error out"=w368:errorcluster)  [unwired: 9 in, 1 out]
            n209 = Release Queue(queue=w370) -> ()  [unwired: 2 in, 3 out]
            n210 = call "CryoCooler Message Log.vi"("String in"="CryoCooler shutting down.") -> ()  [unwired: 9 in, 2 out]
            n211 = call <vilib>:"Clear Errors.vi"("error in (no error)"=w368) -> ()  [unwired: 5 in, 2 out]
          }
        }
      }
      event "Settings Button": Value Change {
        n212 = event-data() -> ()  [unwired: 1 in, 6 out]
        n213 = Unbundle By Name(w382) -> ("PDUs"=w380:refnum<class "Power Distribution.lvclass">[])
        n214 = Select(t=0, s="Settings Button", f=1) -> (s? t:f=w374:i32)
        n215 = Index Array(array=w380, index=w374) -> (element=w381:refnum<class "Power Distribution.lvclass">)
        n216 = call-dynamic "PDU GUI Configure.vi"("Power Distribution in"=w381) -> ("Power Distribution out"=w379:refnum<class "Power Distribution.lvclass">)  [unwired: 9 in, 1 out]
        n217 = Replace Array Subset(array=w380, new element=w379, index=w374) -> (w378:refnum<class "Power Distribution.lvclass">[])
        n218 = Bundle By Name(cluster=w382, "PDUs"=w378) -> (w383:T10)
      }
      event "Refresh Button": Value Change {
        n219 = event-data() -> ()  [unwired: 1 in, 6 out]
        n220 = Unbundle By Name(w397) -> ("PDUs"=w393:refnum<class "Power Distribution.lvclass">[])
        n221 = Select(t=0, s="Refresh Button", f=1) -> (s? t:f=w392:i32)
        n222 = Select(t="Relay Set", s="Refresh Button", f="Relay Set 2") -> (s? t:f=w388:bool[])
        n223 = Index Array(array=w393, index=w392) -> (element=w396:refnum<class "Power Distribution.lvclass">)
        n224 = call-dynamic "PDU Set All Outlets.vi"("State"=w388, "Power Distribution in"=w396) -> ("States out"=w385:bool[], "Power Distribution out"=w386:refnum<class "Power Distribution.lvclass">)  [unwired: 7 in, 1 out]
        n225 = case shown="True" TRUE {
          tunnel: w385 -> [w399 w400]
          frame False {
            n226 = local write "Relay Set 2"(w399) -> ()
          }
          frame True {
            n227 = local write "Relay Set"(w400) -> ()
          }
        }
        n228 = Replace Array Subset(array=w393, new element=w386, index=w392) -> (w391:refnum<class "Power Distribution.lvclass">[])
        n229 = Bundle By Name(cluster=w397, "PDUs"=w391) -> (w398:T10)
      }
      event "Configure Alarms": Value Change {
        n230 = event-data() -> ()  [unwired: 1 in, 6 out]
        n231 = Unbundle By Name(w401) -> ("Cryo Cooler ref"=w406:refnum<class "Cryo Cooler.lvclass">)
        n232 = call-dynamic "Configure Alarms.vi"("Cryo Cooler in"=w406) -> ("error out"=w403:errorcluster, "Cryo Cooler out"=w405:refnum<class "Cryo Cooler.lvclass">)  [unwired: 9 in]
        n233 = call "Rd Wr CryoCooler Alarm Settings.vi"("error in (no error)"=w403) -> ("Cryo Alarms out"=w404:T8)  [unwired: 9 in, 1 out]
        n234 = Bundle By Name(cluster=w401, "Cryo Cooler ref"=w405, "Cryo Alarms"=w404) -> (w402:T10)
      }
      event "Shutdown Temp": Value Change {
        n235 = event-data() -> ()  [unwired: 1 in, 6 out]
        n236 = call "Rd Wr CryoCooler Alarm Settings.vi"() -> ("Cryo Alarms out"=w412:T8)  [unwired: 10 in, 1 out]
        n237 = Bundle By Name(cluster=w412, "Reject Shutdown Temp"="Shutdown Temp") -> (w411:T8)
        n238 = call "Rd Wr CryoCooler Alarm Settings.vi"("Write? (F:Read)"=TRUE, "Cryo Alarms"=w411) -> ("Cryo Alarms out"=w408:T8)  [unwired: 8 in, 1 out]
        n239 = Bundle By Name(cluster=w409, "Cryo Alarms"=w408) -> (w407:T10)
      }
      event "Standalone": Value Change {
        n240 = event-data() -> ("NewVal"=w414:bool)  [unwired: 1 in, 5 out]
        n241 = property on="Close" class="Bool"("Visible"=w414) -> ()  [unwired: 2 in, 2 out]
      }
      event "Status": Value Change {
        n242 = event-data() -> ("NewVal"=w418:i32[])  [unwired: 1 in]
        n243 = call "CC CryoCooler Data buffer.vi"() -> ("XY Graph"=w422:T3)  [unwired: 10 in, 1 out]
        n244 = call "Rd Wr CryoCooler User Interface Settings.vi"() -> ("Settings"=w419:T17)  [unwired: 10 in, 1 out]
        n245 = for {
          tunnel: w418 -> [w427] mode=indexing
          tunnel: w422 -> [w428]
          tunnel: [w426] -> w421 mode=indexing
          n246 = Index Array(array=w428, index=w427) -> (element=w426:T21)
        }
        n247 = Bundle By Name(cluster=w419, "Select Ch"=w418) -> (w417:T17)
        n248 = Unbundle By Name(w425) -> ("Cryo Cooler ref"=w424:refnum<class "Cryo Cooler.lvclass">)
        n249 = property class="Cryo Cooler.lvclass"(reference=w424) -> ("Channels"=w423:string[])  [unwired: 1 in, 2 out]
        n250 = call "Rd Wr CryoCooler User Interface Settings.vi"("Write? (F:Read)"=TRUE, "Settings"=w417) -> ()  [unwired: 8 in, 2 out]
        n251 = property on="XY Graph" class="XYGraph (strict)"("Value"=w421) -> (error out=w420:errorcluster)  [unwired: 2 in, 1 out]
        n252 = for {
          N -> [w430]
          tunnel: w418 -> [w433] mode=indexing
          tunnel: w423 -> [w434]
          tunnel: w420 -> [w429]
          i -> [w432]
          n253 = Index Array(array=w434, index=w433) -> (element=w431:string)
          n254 = property on="XY Graph" class="XYGraph (strict)"(error in=w429, "Active Plot"=w432, "Plot.Plot Name"=w431, "LegNumRows"=w430) -> ()  [unwired: 1 in, 2 out]
        }
      }
      event "CryoCooler Type": Value Change {
        n255 = event-data() -> ("CtlRef"=w442:refnum<vi>)  [unwired: 1 in, 5 out]
        n256 = property class="Ring (strict)"(reference=w442) -> ("Strings []"=w441:string[])  [unwired: 1 in, 2 out]
        n257 = Unbundle By Name(w437) -> ("state"=w436:refnum<user-event>)
        n258 = Generate User Event(user event=w436, event data cluster="Reinit" ("event data")) -> ()  [unwired: 2 in, 2 out]
        n259 = Index Array(array=w441, index="CryoCooler Type") -> (element=w439:string)
        n260 = Bundle By Name(cluster=w437, "Cryo Name"=w439) -> (w438:T10)
      }
      event "Address": Value Change {
        n261 = event-data() -> ()  [unwired: 1 in, 6 out]
        n262 = Unbundle By Name(w451) -> ("state"=w450:refnum<user-event>)  [unwired: 1 out]
        n263 = local read "Select Cryo Cooler"() -> (w447:u16)
        n264 = call "Rd Wr CryoCooler AVC settings json.vi"() -> ("CryoCooler Settings"=w445:T18)  [unwired: 10 in, 1 out]
        n265 = Unbundle By Name(w445) -> ("Cryo Addr"=w448:refnum<visa-resource-name>[])
        n266 = Generate User Event(user event=w450, event data cluster="Reinit" ("event data")) -> ()  [unwired: 2 in, 2 out]
        n267 = Replace Array Subset(array=w448, new element="Address", index=w447) -> (w444:refnum<visa-resource-name>[])
        n268 = Bundle By Name(cluster=w445, "Cryo Addr"=w444) -> (w443:T18)
        n269 = call "Rd Wr CryoCooler AVC settings json.vi"("Write? (F:Read)"=TRUE, "CryoCooler Settings"=w443) -> ()  [unwired: 8 in, 2 out]
      }
      event "Reinit": Value Change {
        n270 = event-data() -> ()  [unwired: 1 in, 6 out]
        n271 = Unbundle By Name(w453) -> ("state"=w455:refnum<user-event>)
        n272 = Generate User Event(user event=w455, event data cluster="Reinit" ("event data")) -> ()  [unwired: 2 in, 2 out]
      }
      event "Execute command": Value Change {
        n273 = event-data() -> ()  [unwired: 1 in, 1 out]
        n274 = Unbundle By Name(w459) -> ("state"=w458:refnum<user-event>)
        n275 = Generate User Event(user event=w458, event data cluster="send command" ("event data")) -> ()  [unwired: 2 in, 2 out]
        n276 = Bundle By Name(cluster=w459, "Cryo Cmd.Cryo Idx"="Select Cryo Cooler", "Cryo Cmd.Command"="Command", "Cryo Cmd.Options"="Command Options") -> (w460:T10)
      }
      event "Select Cryo Cooler": Value Change {
        n277 = event-data() -> ("NewVal"=w464:u16)  [unwired: 1 in]
        n278 = call "Rd Wr CryoCooler AVC settings json.vi"() -> ("CryoCooler Settings"=w466:T18)  [unwired: 10 in, 1 out]
        n279 = Unbundle By Name(w466) -> ("Cryo Addr"=w465:refnum<visa-resource-name>[])
        n280 = Index Array(array=w465, index=w464) -> (element=w463:refnum<visa-resource-name>)
        n281 = local write "Address"(w463) -> ()
      }
      event "Cryo 1 Pwr", "Cryo 2 Pwr": Value Change {
        w482 = T4 1 items=["STATUS", "COOLER", "E", "ERROR", "KD", "KI", "KP", "LOGIN", "LOGOUT", "MODE", "P", "PWOUT", "SENSOR", "TC", "TEMP RJ", "TTARGET", "VERSION"] ("Cryo Cmd.Command")
        n282 = event-data() -> ("CtlRef"=w475:refnum<vi>)  [unwired: 1 in]
        n283 = property class="Bool (strict)"(reference=w475) -> ("Label.Text"=w478:string)  [unwired: 1 in, 2 out]
        n284 = Unbundle By Name(w473) -> ("state"=w484:refnum<user-event>)
        n285 = Match Pattern(string=w478, regular expression=".*2") -> (offset past match=w476:i32)  [unwired: 1 in, 3 out]
        n286 = Less Than 0?(x=w476) -> (x < 0?=w472:bool)
        n287 = Generate User Event(user event=w484, event data cluster="send command" ("event data")) -> ()  [unwired: 2 in, 2 out]
        n288 = case shown="False" w472 {
          tunnel: "Cryo 1 Pwr" -> [_ w488]
          tunnel: [w486 w488] -> w470
          tunnel: [1 0] -> w469
          tunnel: "Cryo 2 Pwr" -> [w486 _]
          frame False {
          }
          frame True {
          }
        }
        n289 = Select(t="On", s=w470, f="Off") -> (s? t:f=w479:string)
        n290 = Bundle By Name(cluster=w473, "Cryo Cmd.Command"=w482, "Cryo Cmd.Options"=w479, "Cryo Cmd.Cryo Idx"=w469) -> (w474:T10)
      }
      event Value Change {
        n291 = event-data() -> ()  [unwired: 1 in, 6 out]
        n292 = case shown="\"User\", Default" "Mode" {
          tunnel: [bool[] [TRUE, FALSE, FALSE] bool[] [TRUE, TRUE, TRUE]] -> w489
          frame "User", Default {
          }
          frame "Engineering" {
          }
        }
        n293 = property on="Tab Control" class="TabCtl (strict)"() -> ("Pages"=w490:refnum<vi>[])  [unwired: 2 in, 2 out]
        n294 = for {
          tunnel: w490 -> [w494] mode=indexing
          tunnel: w489 -> [w493] mode=indexing
          n295 = property class="Page"(reference=w494, "PageVis"=w493) -> ()  [unwired: 1 in, 2 out]
        }
      }
      event "Close": Value Change {
        n296 = event-data() -> ()  [unwired: 1 in, 2 out]
        n297 = Unbundle By Name(w499) -> ("state"=w498:refnum<user-event>)
        n298 = Generate User Event(user event=w498, event data cluster="Shutdown" ("event data")) -> ()  [unwired: 2 in, 2 out]
      }
    }
  }
